vi "AllContexts.vi"(11 "error in (no error)":errorcluster) -> (4 "Context[]":string[](array[string]), 6 "Project[]":string[](array[string]), 8 "ProjectPath[]":path[](array[path]), 15 "error out":errorcluster)   [LabVIEW 2016, in "LabVIEWCodeCoverage.lvlib"]
uses:
  LabVIEWCodeCoverage.lvlib
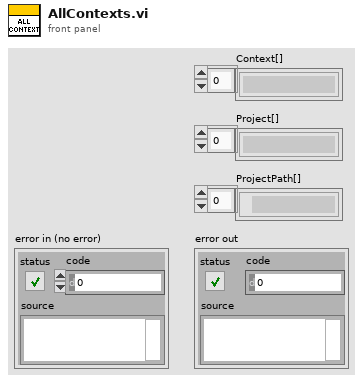
[diagram p1: front panel]
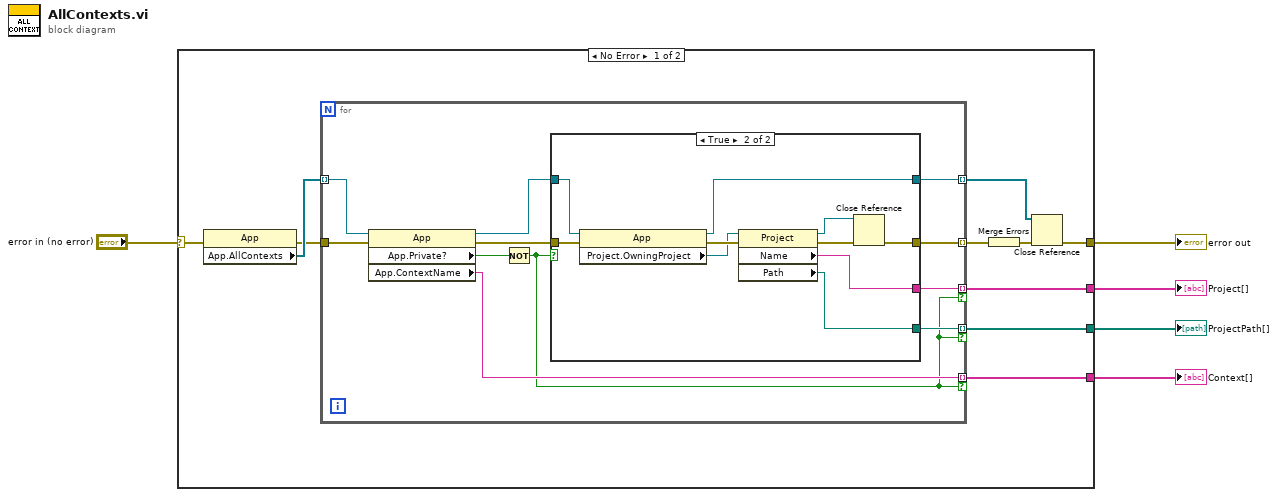
[diagram p0: block diagram]
diagram:
  n1 = case shown="No Error" "error in (no error)" {
    selector: "error in (no error)" -> [w12 w39]
    tunnel: [w9 _] -> w4
    tunnel: [w8 w39] -> w3
    tunnel: [w7 _] -> w2
    tunnel: [w6 _] -> w1
    frame No Error {
      n2 = property class="App"(error in=w12) -> (error out=w13:errorcluster, "App.AllContexts"=w15:refnum<vi>[])  [unwired: 1 in, 1 out]
      n3 = for {
        tunnel: w15 -> [w25] mode=indexing
        tunnel: [w20] -> w10 mode=indexing
        tunnel: w13 -> [w26]
        tunnel: [w22] -> w14 mode=indexing
        tunnel: [w19] -> w9 mode=indexing if=w16
        tunnel: [w18] -> w7 mode=indexing if=w16
        tunnel: [w17] -> w6 mode=indexing if=w16
        n4 = property class="App"(reference=w25, error in=w26) -> (reference out=w21:refnum<vi>, error out=w24:errorcluster, "App.Private?"=w23:bool, "App.ContextName"=w18:string)
        n5 = Not(x=w23) -> (.not. x?=w16:bool)
        n6 = case shown="True" w16 {
          tunnel: w21 -> [w27 w34]
          tunnel: [_ w38] -> w19
          tunnel: w24 -> [w28 w35]
          tunnel: [w28 w32] -> w22
          tunnel: [w27 w30] -> w20
          tunnel: [_ w29] -> w17
          frame False {
          }
          frame True {
            n7 = property class="App"(reference=w34, error in=w35) -> (reference out=w30:refnum<vi>, error out=w36:errorcluster, "Project.OwningProject"=w33:refnum<vi>)
            n8 = property class="Project"(reference=w33, error in=w36) -> (reference out=w31:refnum<vi>, error out=w37:errorcluster, "Name"=w38:string, "Path"=w29:path)
            n9 = Close Reference(reference=w31, error in (no error)=w37) -> (error out=w32:errorcluster)
          }
        }
      }
      n10 = Merge Errors(w14) -> (w11:errorcluster)
      n11 = Close Reference(reference=w10, error in (no error)=w11) -> (error out=w8:errorcluster)
    }
    frame Error {
    }
  }
  "Project[]" <- w4
  "error out" <- w3
  "Context[]" <- w2
  "ProjectPath[]" <- w1
